vi "AlGaInPAs_v22a.vi"(2 "Debug Mode":bool, 3 "Elapsed Time(s)":dbl, 4 "State":enum16{"Edit", "Start", "Run", "End", "Idle"}(ring), 5 "Argument List In":string[](array[string])) -> (0 "Status Out":string, 1 "Argument List Out":string[](array[string]))   [LabVIEW 2011]
uses:
  high_level_proc/source_dilution.ctl
  high_level_proc/source_noDilution.ctl
panel:
  out "source array":refnum<vi>[](array[refnum])
  in  "Zn bubbler":T1={"Dilution"=FALSE, "Calculated"=0, "MFC1 flow"=0.0, "MFC2 flow"=10.0, "MFC3 flow"=100.0, "Bubbler (main)"={"Flow"=0.0, "Prep"=FALSE, "Run"=FALSE, "Active"=FALSE, "Name"=""}} caption="Al" {"Bubbler (main)"."Flow" format="%.2f"; "MFC1 flow" format="%.4f"; "MFC3 flow" format="%.1f"; "MFC2 flow" format="%.2f"; "Calculated" items=["Flow", "MFC1", "MFC2", "MFC3"]}
  in  "Al bubbler":T2 caption="Al" {"Flow" format="%.2f"}
  in  "Se bubbler":T1={"Dilution"=FALSE, "Calculated"=0, "MFC1 flow"=0.0, "MFC2 flow"=10.0, "MFC3 flow"=100.0, "Bubbler (main)"={"Flow"=0.0, "Prep"=FALSE, "Run"=FALSE, "Active"=FALSE, "Name"="Se"}} caption="Al" {"Bubbler (main)"."Flow" format="%.2f"; "MFC1 flow" format="%.4f"; "MFC3 flow" format="%.1f"; "MFC2 flow" format="%.2f"; "Calculated" items=["Flow", "MFC1", "MFC2", "MFC3"]}
  in  "P bubbler":T2={"Flow"=0.0, "Prep"=FALSE, "Run"=FALSE, "Active"=FALSE, "Name"="P liq"} caption="Al" {"Flow" format="%.2f"}
  in  "As gas":T2={"Flow"=0.0, "Prep"=FALSE, "Run"=FALSE, "Active"=FALSE, "Name"="As gas"} caption="Al" {"Flow" format="%.2f"}
  in  "P gas":T2={"Flow"=0.0, "Prep"=FALSE, "Run"=FALSE, "Active"=FALSE, "Name"="P gas"} caption="Al" {"Flow" format="%.2f"}
  in  "In bubbler":T2 caption="Al" {"Flow" format="%.2f"}
  in  "Ga bubbler":T1={"Dilution"=FALSE, "Calculated"=0, "MFC1 flow"=0.0, "MFC2 flow"=10.0, "MFC3 flow"=100.0, "Bubbler (main)"={"Flow"=0.0, "Prep"=FALSE, "Run"=FALSE, "Active"=FALSE, "Name"=""}} caption="Al" {"Bubbler (main)"."Flow" format="%.2f"; "MFC1 flow" format="%.4f"; "MFC3 flow" format="%.1f"; "MFC2 flow" format="%.2f"; "Calculated" items=["Flow", "MFC1", "MFC2", "MFC3"]}
  out "prep_done":bool
  out "run started":bool
  out "first":bool=TRUE
  out "is OK?":bool
  in  "prep_time":dbl
  in  "Cancel":bool
  in  "OK":bool
  # "s"
  # "Add pre-run time to run time in editor."
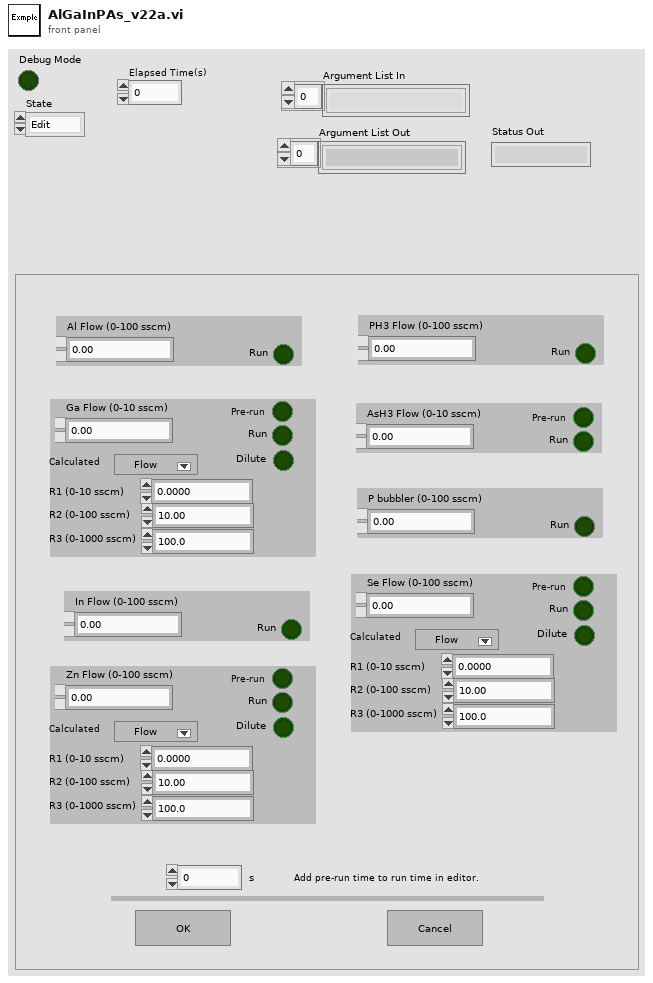
[diagram p1: front panel]
types:
  T1 = typedef "source_dilution.ctl" = cluster{"Dilution":bool, "Calculated":u16, "MFC1 flow":dbl, "MFC2 flow":dbl, "MFC3 flow":dbl, "Bubbler (main)":T2}
  T2 = typedef "source_noDilution.ctl" = cluster{"Flow":dbl, "Prep":bool, "Run":bool, "Active":bool, "Name":string}
  T3 = enum32{"Invalid", "Default", "Floating", "Floating/Auto-Hide", "Modal"}
  T4 = enum16{"Discrete", "Continuous", "Instantaneous", "Finite"}
  T5 = cluster{"Flow":dbl, "Prep":bool, "Run":bool, "Active":bool, "Name":string}
  T6 = cluster{"Dilution":bool, "Calculated":u16, "MFC1 flow":dbl, "MFC2 flow":dbl, "MFC3 flow":dbl, "Bubbler (main)":T2}
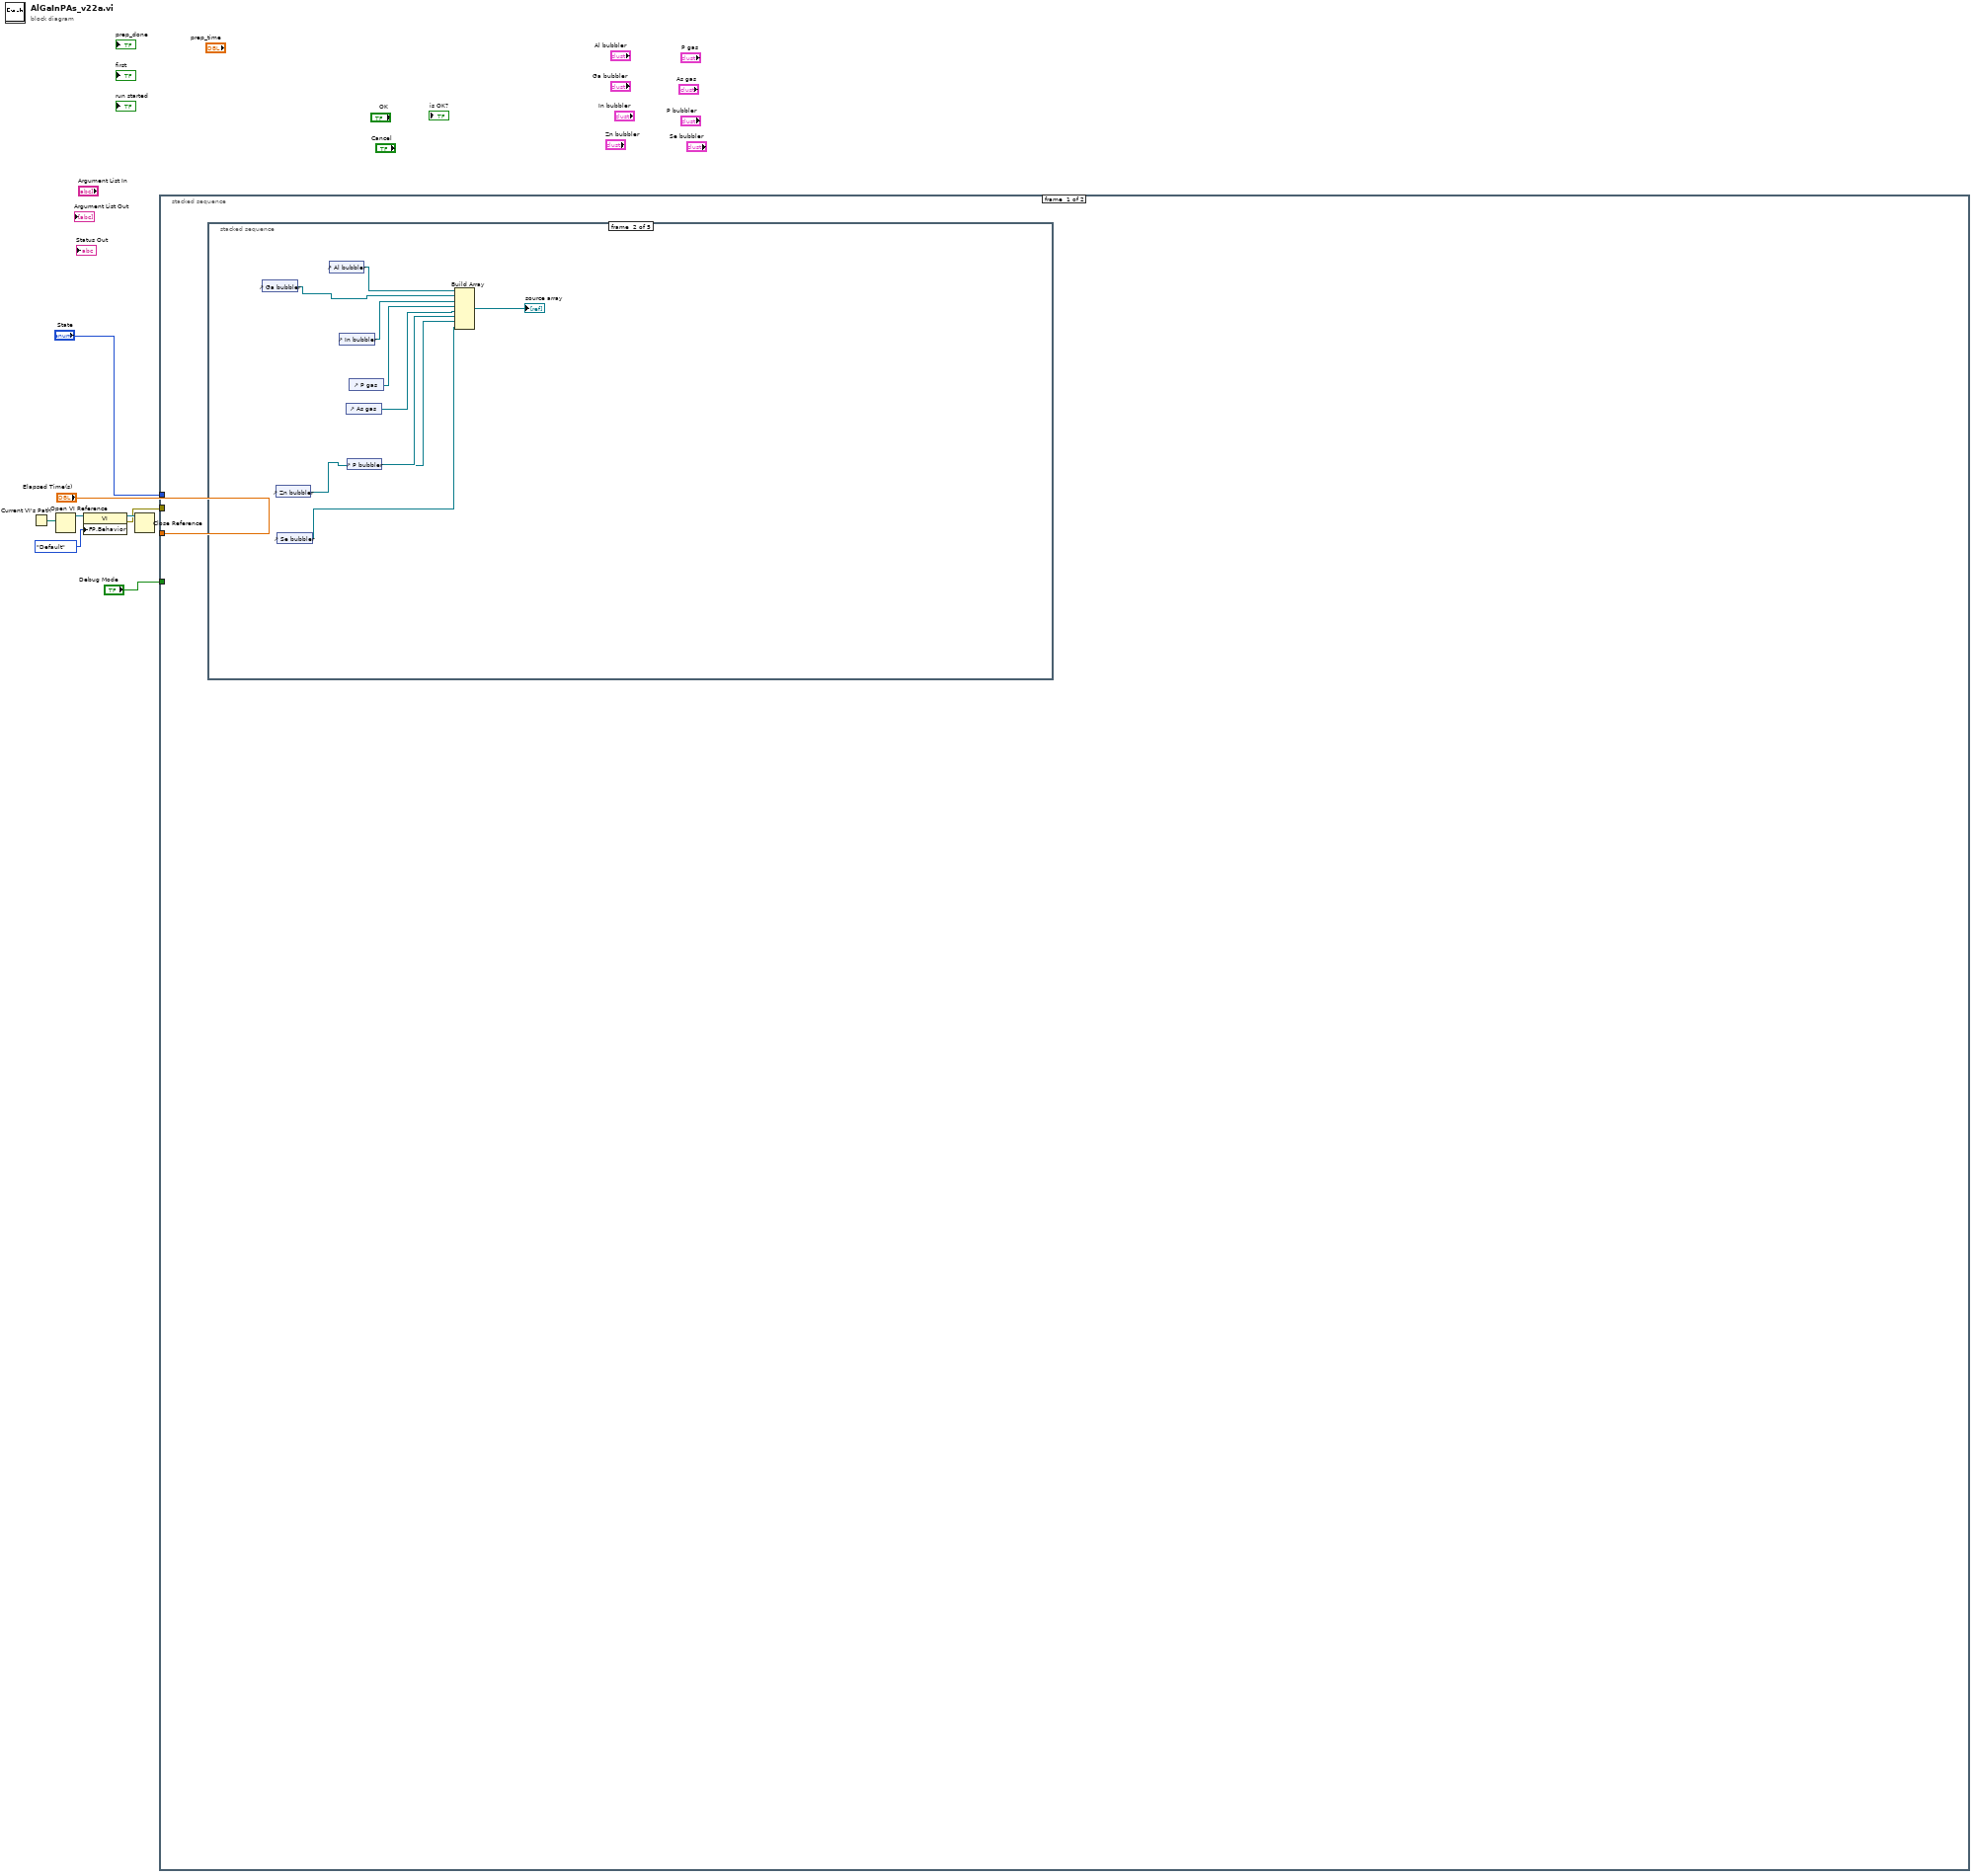
[diagram p0: block diagram]
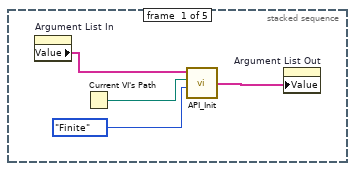
[diagram p2: hidden frame]
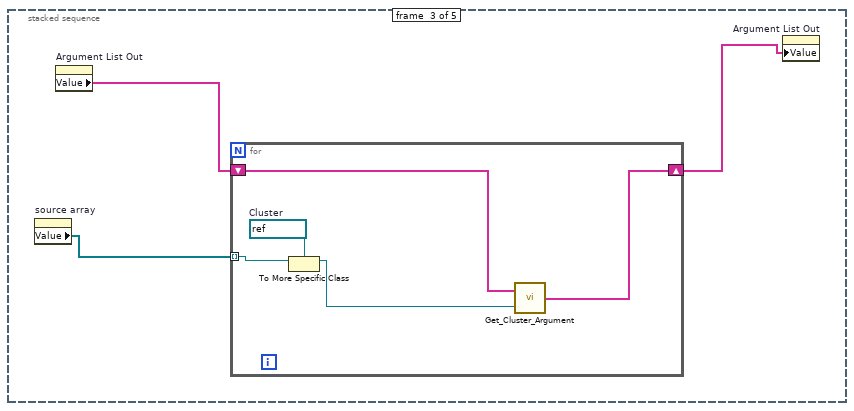
[diagram p3: hidden frame]
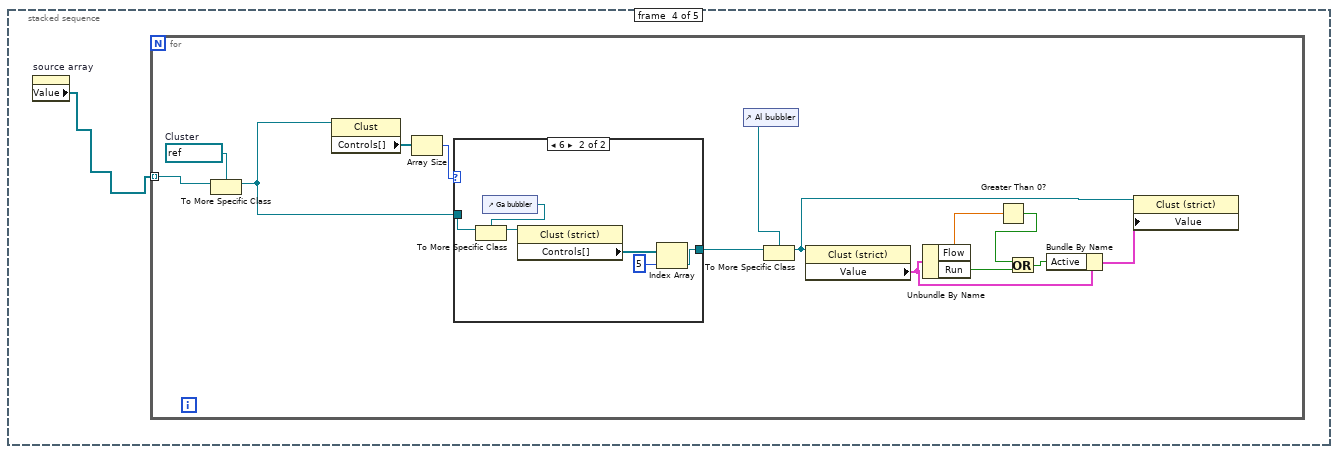
[diagram p4: hidden frame]
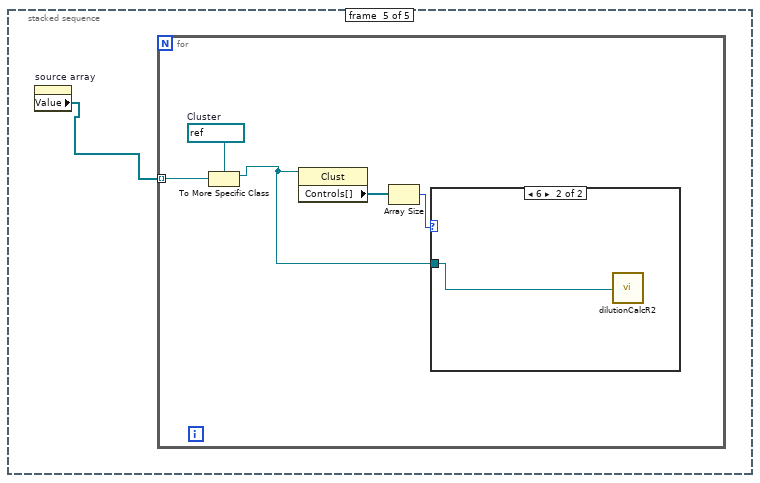
[diagram p6: hidden frame]
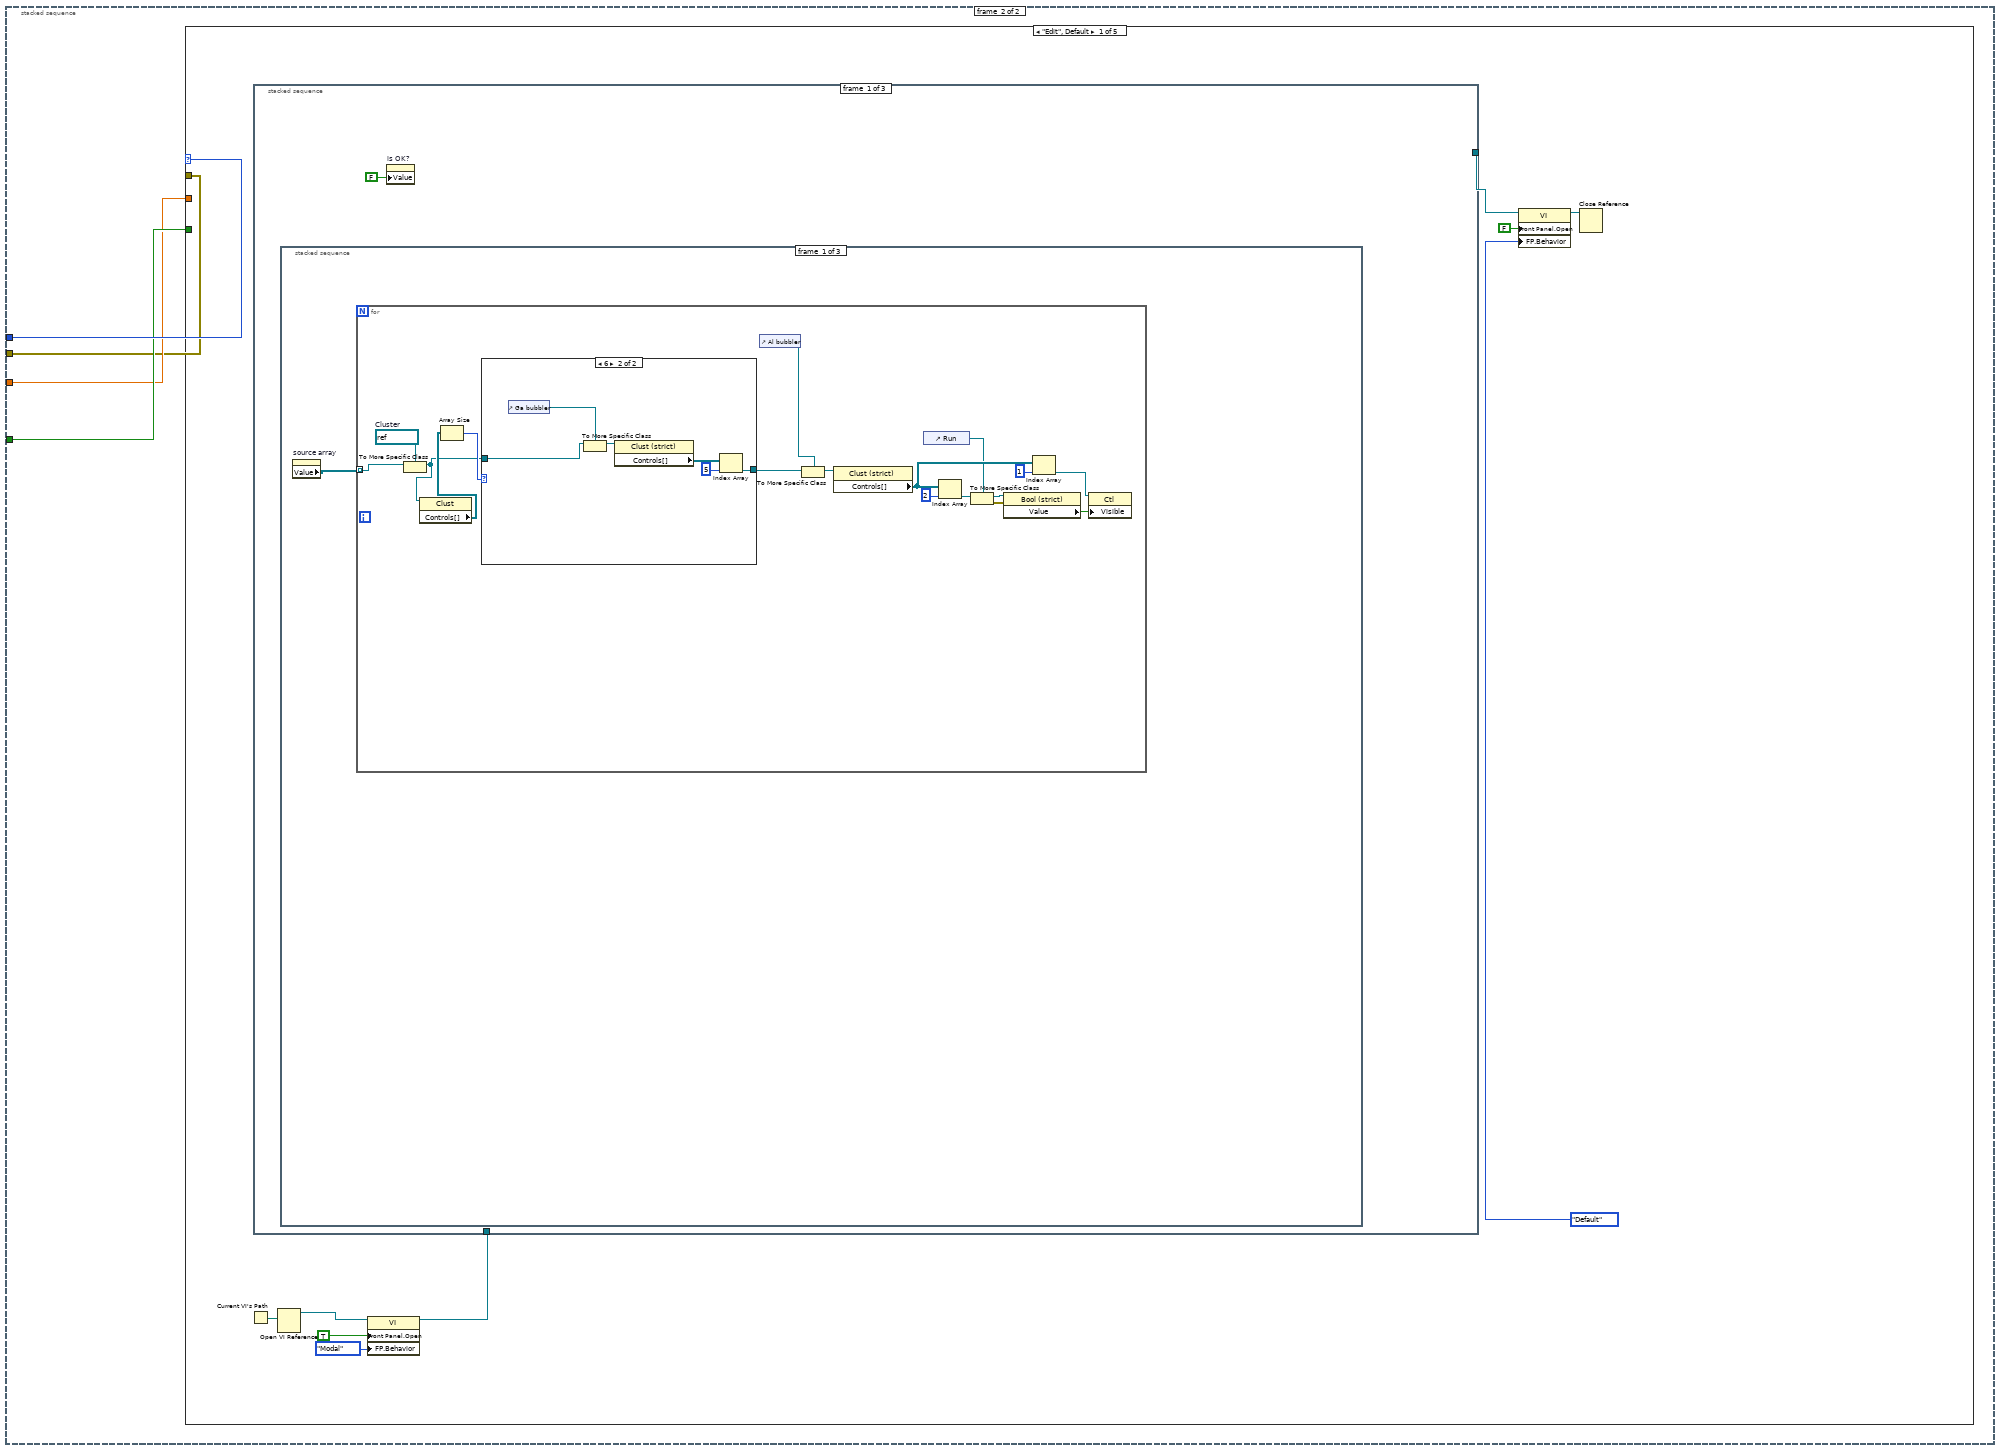
[diagram p8: hidden frame]
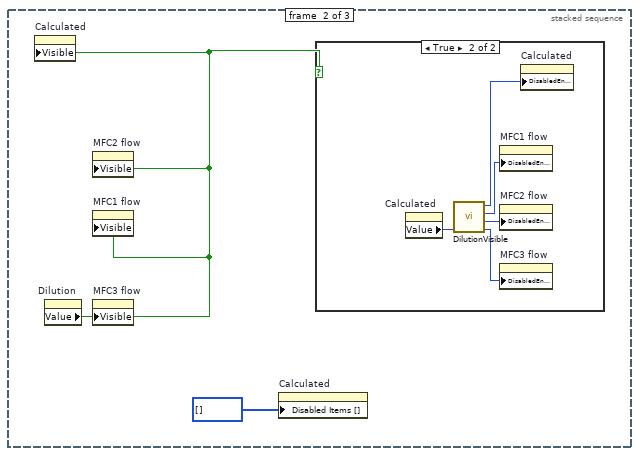
[diagram p10: hidden frame]
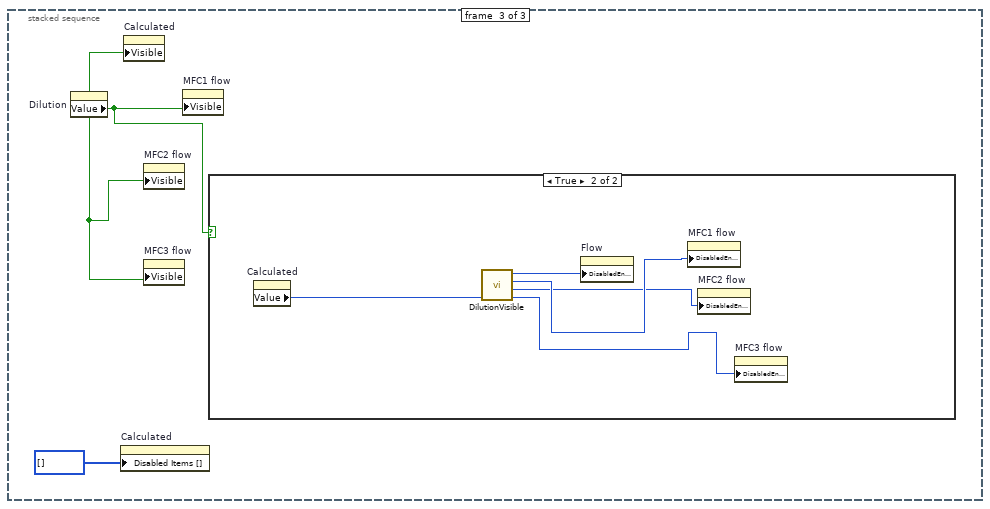
[diagram p12: hidden frame]
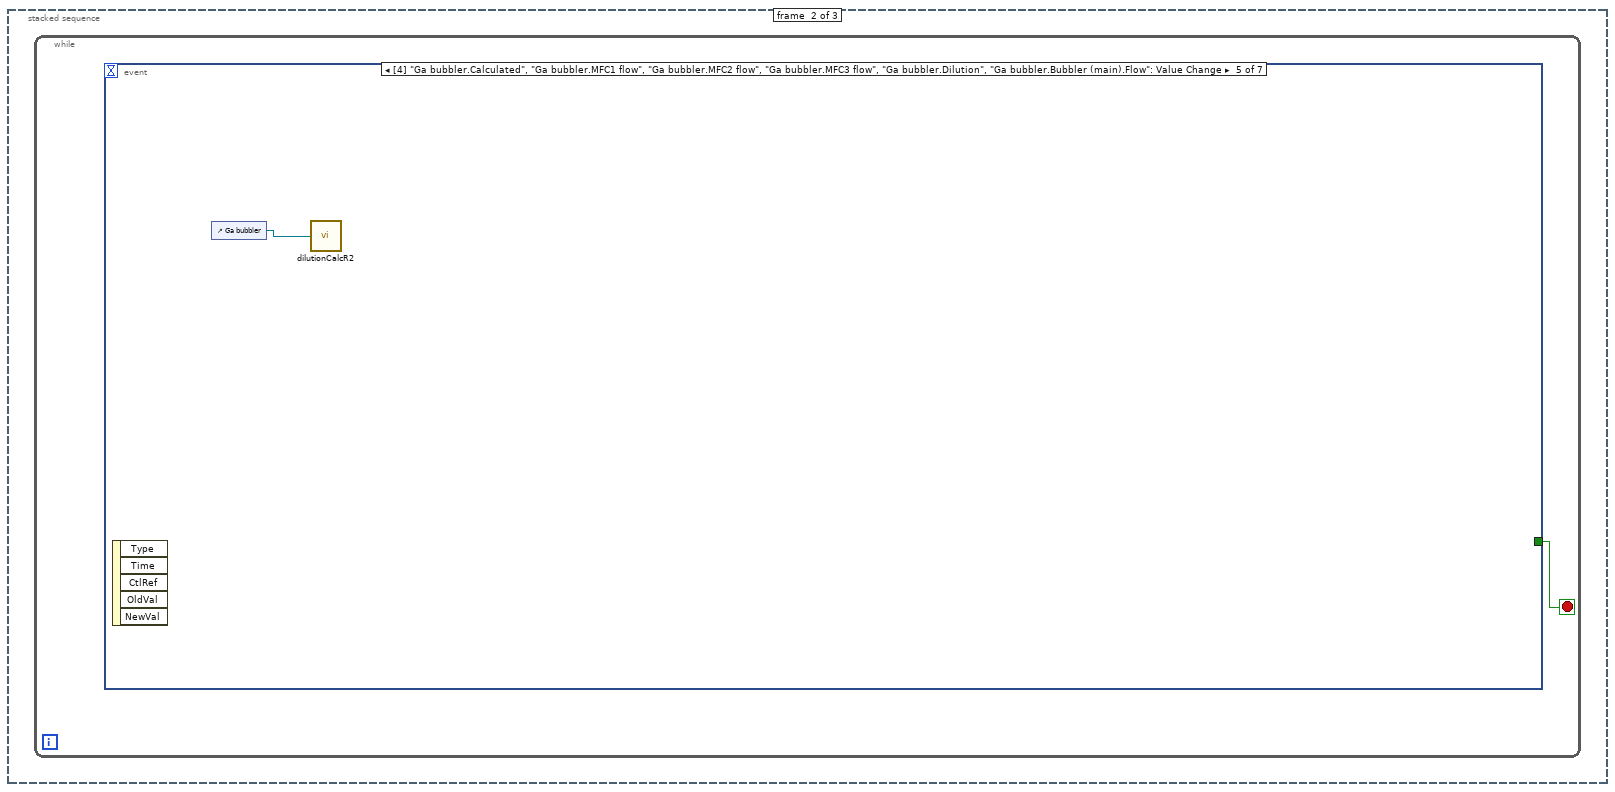
[diagram p14: hidden frame]
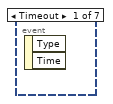
[diagram p15: hidden frame]
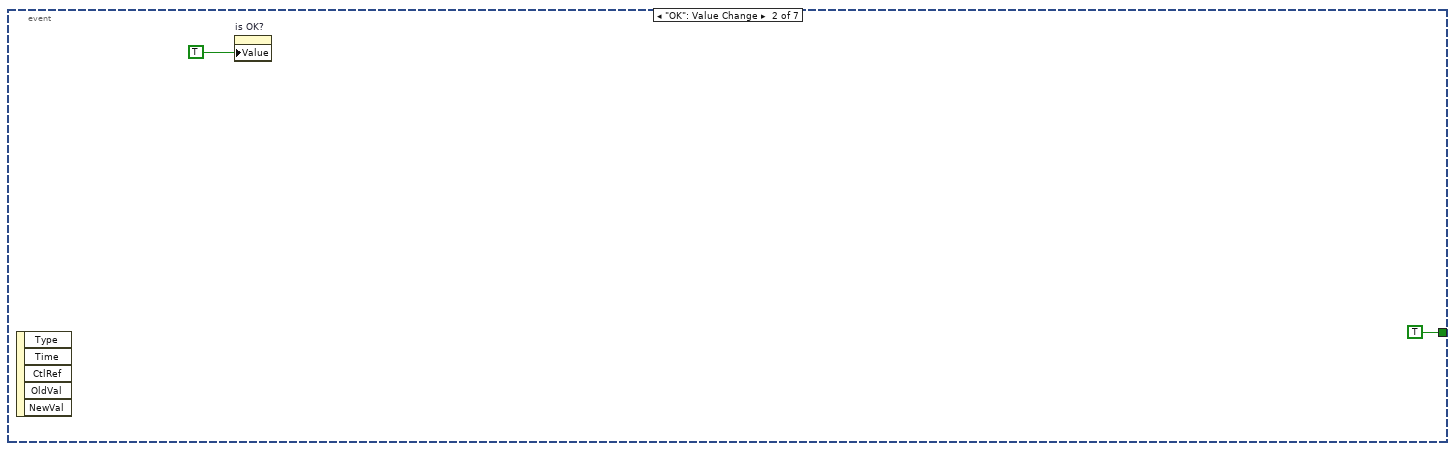
[diagram p16: hidden frame]
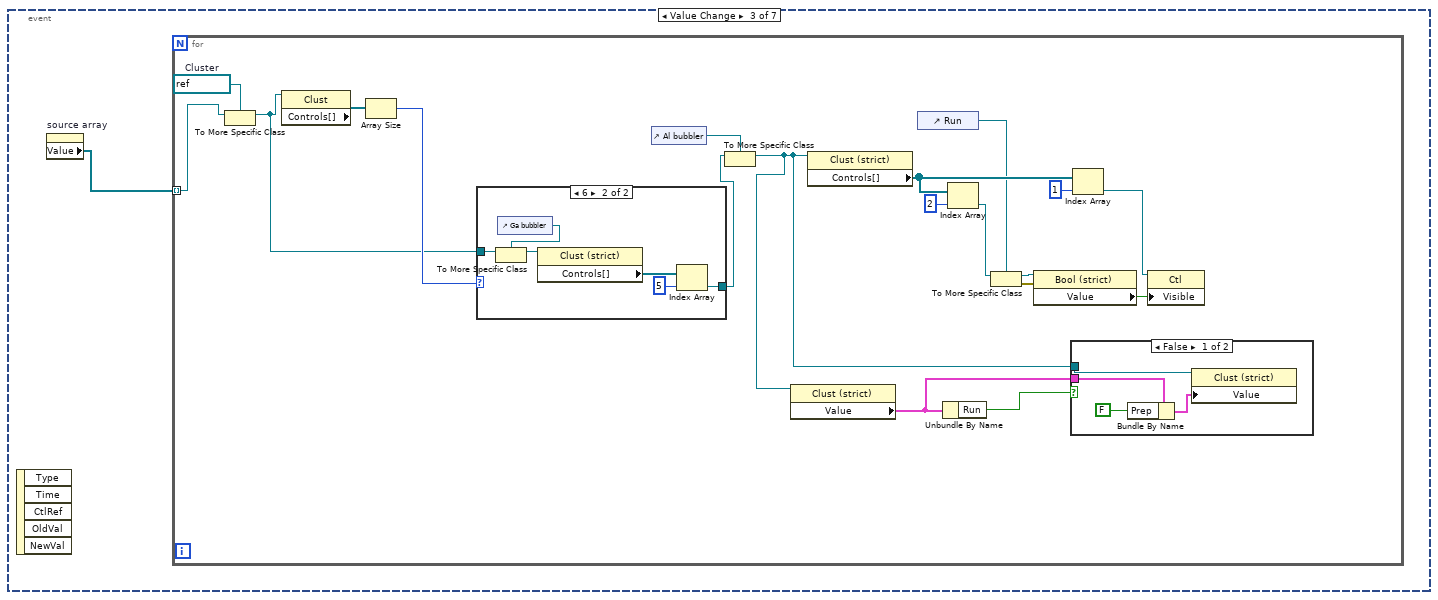
[diagram p17: hidden frame]
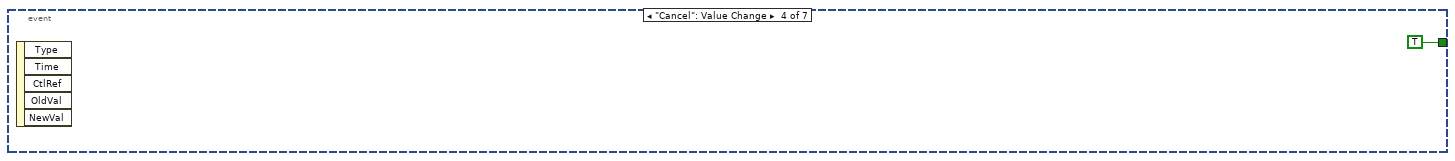
[diagram p20: hidden frame]
diagram:
  n1 = Current VI's Path() -> (path=w5:path)
  n2 = Open VI Reference(vi path=w5) -> (vi reference=w4:refnum<vi>)  [unwired: 1 in, 5 out]
  n3 = property class="VI"(reference=w4, "FP.Behavior"=T3."Default" ("Front Panel Window:Behavior")) -> (reference out=w2:refnum<vi>, error out=w1:errorcluster)  [unwired: 1 in]
  n4 = Close Reference(reference=w2) -> ()  [unwired: 1 in, 1 out]
  n5 = stacked-sequence {
    tunnel: "State" -> [_ w62]
    tunnel: "Debug Mode" -> [_ w61]
    tunnel: "Elapsed Time(s)" -> [_ w60]
    tunnel: w1 -> [_ w59]
    frame #0 {
      n6 = stacked-sequence {
        frame #0 {
          n7 = property on="Argument List In" class="Arr (strict)"() -> ("Value"=w12:string[])  [unwired: 2 in, 2 out]
          n8 = Current VI's Path() -> (path=w9:path)
          n9 = call "API_Init.vi"("API Mode"=T4."Finite", "VI Path"=w9, "Argument List In"=w12) -> ("Argument List Out"=w11:string[])  [unwired: 1 in]
          n10 = property on="Argument List Out" class="Arr (strict)"("Value"=w11) -> ()  [unwired: 2 in, 2 out]
        }
        frame #1 {
          n11 = control-ref of="Ga bubbler"() -> (w16:refnum<vi>)
          n12 = control-ref of="Zn bubbler"() -> (w15:refnum<vi>)
          n13 = control-ref of="Se bubbler"() -> (w14:refnum<vi>)
          n14 = control-ref of="Al bubbler"() -> (w21:refnum<vi>)
          n15 = control-ref of="In bubbler"() -> (w20:refnum<vi>)
          n16 = control-ref of="As gas"() -> (w18:refnum<vi>)
          n17 = control-ref of="P bubbler"() -> (w17:refnum<vi>)
          n18 = control-ref of="P gas"() -> (w19:refnum<vi>)
          n19 = Build Array(w21, w16, w20, w19, w18, w17, w15, w14) -> (→"source array":refnum<vi>[])
        }
        frame #2 {
          n20 = property on="source array" class="Arr (strict)"() -> ("Value"=w22:refnum<vi>[])  [unwired: 2 in, 2 out]
          n21 = property on="Argument List Out" class="Arr (strict)"() -> ("Value"=w24:string[])  [unwired: 2 in, 2 out]
          n22 = for {
            shift-right: [w28] -> w23
            shift-left: w24 -> [w29]
            tunnel: w22 -> [w27] mode=indexing
            w25 = refnum<vi> refnum  # Cluster
            n23 = To More Specific Class(target class=w25, reference=w27) -> (specific class reference=w26:refnum<vi>)  [unwired: 1 in, 1 out]
            n24 = call "Get_Cluster_Argument.vi"("source"=w26, "Argument List In"=w29) -> ("Argument List Out"=w28:string[])
          }
          n25 = property on="Argument List Out" class="Arr (strict)"("Value"=w23) -> ()  [unwired: 2 in, 2 out]
        }
        frame #3 {
          n26 = property on="source array" class="Arr (strict)"() -> ("Value"=w30:refnum<vi>[])  [unwired: 2 in, 2 out]
          n27 = for {
            tunnel: w30 -> [w33] mode=indexing
            w31 = refnum<vi> refnum  # Cluster
            n28 = To More Specific Class(target class=w31, reference=w33) -> (specific class reference=w32:refnum<vi>)  [unwired: 1 in, 1 out]
            n29 = property class="Clust"(reference=w32) -> ("Controls[]"=w35:refnum<vi>[])  [unwired: 1 in, 2 out]
            n30 = Array Size(array=w35) -> (size(s)=w36:i32)
            n31 = case shown="6" w36 {
              tunnel: [w45 w47] -> w34
              tunnel: w32 -> [w45 w50]
              frame Default {
              }
              frame 6 {
                n32 = control-ref of="Ga bubbler"() -> (w46:refnum<vi>)
                n33 = To More Specific Class(target class=w46, reference=w50) -> (specific class reference=w49:refnum<vi>)  [unwired: 1 in, 1 out]
                n34 = property class="Clust (strict)"(reference=w49) -> ("Controls[]"=w48:refnum<vi>[])  [unwired: 1 in, 2 out]
                n35 = Index Array(array=w48, index=5) -> (element=w47:refnum<vi>)
              }
            }
            n36 = control-ref of="Al bubbler"() -> (w38:refnum<vi>)
            n37 = To More Specific Class(target class=w38, reference=w34) -> (specific class reference=w37:refnum<vi>)  [unwired: 1 in, 1 out]
            n38 = property class="Clust (strict)"(reference=w37) -> ("Value"=w41:T5)  [unwired: 1 in, 2 out]
            n39 = Unbundle By Name(w41) -> ("Flow"=w44:dbl, "Run"=w42:bool)
            n40 = Greater Than 0?(x=w44) -> (x > 0?=w43:bool)
            n41 = Or(x=w43, y=w42) -> (x .or. y?=w39:bool)
            n42 = Bundle By Name(cluster=w41, "Active"=w39) -> (w40:T5)
            n43 = property class="Clust (strict)"(reference=w37, "Value"=w40) -> ()  [unwired: 1 in, 2 out]
          }
        }
        frame #4 {
          n44 = property on="source array" class="Arr (strict)"() -> ("Value"=w52:refnum<vi>[])  [unwired: 2 in, 2 out]
          n45 = for {
            tunnel: w52 -> [w56] mode=indexing
            w54 = refnum<vi> refnum  # Cluster
            n46 = To More Specific Class(target class=w54, reference=w56) -> (specific class reference=w55:refnum<vi>)  [unwired: 1 in, 1 out]
            n47 = property class="Clust"(reference=w55) -> ("Controls[]"=w53:refnum<vi>[])  [unwired: 1 in, 2 out]
            n48 = Array Size(array=w53) -> (size(s)=w57:i32)
            n49 = case shown="6" w57 {
              tunnel: w55 -> [_ w58]
              frame Default {
              }
              frame 6 {
                n50 = call "dilutionCalcR2.vi"("Clust Refnum"=w58) -> ()
              }
            }
          }
        }
      }
    }
    frame #1 {
      n51 = case shown="\"Edit\", Default" w62 {
        tunnel: w61 -> [_ w169 w185 _ _]
        tunnel: w60 -> [_ _ w186 _ _]
        tunnel: w59 -> [_ _ _ _ _]
        frame "Edit", Default {
          n52 = Current VI's Path() -> (path=w67:path)
          n53 = Open VI Reference(vi path=w67) -> (vi reference=w66:refnum<vi>)  [unwired: 1 in, 5 out]
          n54 = property class="VI"(reference=w66, "Front Panel.Open"=TRUE ("Front Panel Window:Open"), "FP.Behavior"=T3."Modal" ("Front Panel Window:Behavior")) -> (reference out=w64:refnum<vi>)  [unwired: 1 in, 1 out]
          n55 = stacked-sequence {
            tunnel: [_ _ w152] -> w69
            tunnel: w64 -> [_ _ w152]
            frame #0 {
              n56 = stacked-sequence {
                frame #0 {
                  n57 = property on="source array" class="Arr (strict)"() -> ("Value"=w73:refnum<vi>[])  [unwired: 2 in, 2 out]
                  n58 = for {
                    tunnel: w73 -> [w78] mode=indexing
                    w77 = refnum<vi> refnum  # Cluster
                    n59 = To More Specific Class(target class=w77, reference=w78) -> (specific class reference=w74:refnum<vi>)  [unwired: 1 in, 1 out]
                    n60 = property class="Clust"(reference=w74) -> ("Controls[]"=w76:refnum<vi>[])  [unwired: 1 in, 2 out]
                    n61 = Array Size(array=w76) -> (size(s)=w75:i32)
                    n62 = case shown="6" w75 {
                      tunnel: w74 -> [w91 w94]
                      tunnel: [w91 w95] -> w80
                      frame Default {
                      }
                      frame 6 {
                        n63 = control-ref of="Ga bubbler"() -> (w92:refnum<vi>)
                        n64 = To More Specific Class(target class=w92, reference=w94) -> (specific class reference=w93:refnum<vi>)  [unwired: 1 in, 1 out]
                        n65 = property class="Clust (strict)"(reference=w93) -> ("Controls[]"=w97:refnum<vi>[])  [unwired: 1 in, 2 out]
                        n66 = Index Array(array=w97, index=5) -> (element=w95:refnum<vi>)
                      }
                    }
                    n67 = control-ref of="Al bubbler"() -> (w81:refnum<vi>)
                    n68 = To More Specific Class(target class=w81, reference=w80) -> (specific class reference=w88:refnum<vi>)  [unwired: 1 in, 1 out]
                    n69 = property class="Clust (strict)"(reference=w88) -> ("Controls[]"=w87:refnum<vi>[])  [unwired: 1 in, 2 out]
                    n70 = control-ref of="Run"() -> (w79:refnum<vi>)
                    n71 = Index Array(array=w87, index=2) -> (element=w85:refnum<vi>)
                    n72 = To More Specific Class(target class=w79, reference=w85) -> (specific class reference=w84:refnum<vi>, error out=w83:errorcluster)  [unwired: 1 in]
                    n73 = property class="Bool (strict)"(reference=w84, error in=w83) -> ("Value"=w82:bool)  [unwired: 2 out]
                    n74 = Index Array(array=w87, index=1) -> (element=w89:refnum<vi>)
                    n75 = property class="Ctl"(reference=w89, "Visible"=w82) -> ()  [unwired: 1 in, 2 out]
                  }
                }
                frame #1 {
                  n76 = property on="Dilution" class="Bool (strict)"() -> ("Value"=w99:bool)  [unwired: 2 in, 2 out]
                  n77 = property on="Calculated" class="Ring (strict)"("Visible"=w99) -> ()  [unwired: 2 in, 2 out]
                  n78 = property on="MFC2 flow" class="DigNum (strict)"("Visible"=w99) -> ()  [unwired: 2 in, 2 out]
                  n79 = property on="MFC1 flow" class="DigNum (strict)"("Visible"=w99) -> ()  [unwired: 2 in, 2 out]
                  n80 = property on="MFC3 flow" class="DigNum (strict)"("Visible"=w99) -> ()  [unwired: 2 in, 2 out]
                  n81 = property on="Calculated" class="Ring (strict)"("Disabled Items []"=i32[] []) -> ()  [unwired: 2 in, 2 out]
                  n82 = case shown="True" w99 {
                    frame False {
                    }
                    frame True {
                      n83 = property on="Calculated" class="Ring (strict)"() -> ("Value"=w101:u16)  [unwired: 2 in, 2 out]
                      n84 = call "DilutionVisible.vi"("calculated"=w101) -> ("MFC3"=w104:u16, "MFC2"=w103:u16, "MFC1"=w102:u16, "flow"=w100:u16)  [unwired: 3 in]
                      n85 = property on="MFC1 flow" class="DigNum (strict)"("DisabledEnum"=w102) -> ()  [unwired: 2 in, 2 out]
                      n86 = property on="MFC2 flow" class="DigNum (strict)"("DisabledEnum"=w103) -> ()  [unwired: 2 in, 2 out]
                      n87 = property on="MFC3 flow" class="DigNum (strict)"("DisabledEnum"=w104) -> ()  [unwired: 2 in, 2 out]
                      n88 = property on="Calculated" class="Ring (strict)"("DisabledEnum"=w100) -> ()  [unwired: 2 in, 2 out]
                    }
                  }
                }
                frame #2 {
                  n89 = property on="Dilution" class="Bool (strict)"() -> ("Value"=w105:bool)  [unwired: 2 in, 2 out]
                  n90 = property on="Calculated" class="Ring (strict)"("Disabled Items []"=i32[] []) -> ()  [unwired: 2 in, 2 out]
                  n91 = property on="Calculated" class="Ring (strict)"("Visible"=w105) -> ()  [unwired: 2 in, 2 out]
                  n92 = property on="MFC2 flow" class="DigNum (strict)"("Visible"=w105) -> ()  [unwired: 2 in, 2 out]
                  n93 = property on="MFC3 flow" class="DigNum (strict)"("Visible"=w105) -> ()  [unwired: 2 in, 2 out]
                  n94 = property on="MFC1 flow" class="DigNum (strict)"("Visible"=w105) -> ()  [unwired: 2 in, 2 out]
                  n95 = case shown="True" w105 {
                    frame False {
                    }
                    frame True {
                      n96 = property on="Calculated" class="Ring (strict)"() -> ("Value"=w110:u16)  [unwired: 2 in, 2 out]
                      n97 = call "DilutionVisible.vi"("calculated"=w110) -> ("MFC3"=w108:u16, "MFC2"=w107:u16, "MFC1"=w109:u16, "flow"=w111:u16)  [unwired: 3 in]
                      n98 = property on="Flow" class="DigNum (strict)"("DisabledEnum"=w111) -> ()  [unwired: 2 in, 2 out]
                      n99 = property on="MFC1 flow" class="DigNum (strict)"("DisabledEnum"=w109) -> ()  [unwired: 2 in, 2 out]
                      n100 = property on="MFC2 flow" class="DigNum (strict)"("DisabledEnum"=w107) -> ()  [unwired: 2 in, 2 out]
                      n101 = property on="MFC3 flow" class="DigNum (strict)"("DisabledEnum"=w108) -> ()  [unwired: 2 in, 2 out]
                    }
                  }
                }
              }
              n102 = property on="is OK?" class="Bool (strict)"("Value"=FALSE ("is OK?")) -> ()  [unwired: 2 in, 2 out]
            }
            frame #1 {
              n103 = while {
                stop <- w112 stop-if-true
                n104 = event shown="[4] \"Ga bubbler.Calculated\", \"Ga bubbler.MFC1 flow\", \"Ga bubbler.MFC2 flow\", \"Ga bubbler.MFC3 flow\", \"Ga bubbler.Dilution\", \"Ga bubbler.Bubbler (main).Flow\": Value Change" {
                  selector: _ -> [_ _ _ _ _ _ _]
                  dyn-events: _ -> [_ _ _ _ _ _ _]
                  timeout: _ -> [_ _ _ _ _ _ _]
                  tunnel: [_ TRUE _ TRUE _ _ _] -> w112
                  event Timeout {
                    n105 = event-data() -> ()  [unwired: 1 in, 2 out]
                  }
                  event "OK": Value Change {
                    n106 = event-data() -> ()  [unwired: 1 in, 5 out]
                    n107 = property on="is OK?" class="Bool (strict)"("Value"=TRUE ("is OK?")) -> ()  [unwired: 2 in, 2 out]
                  }
                  event Value Change {
                    n108 = event-data() -> ()  [unwired: 1 in, 5 out]
                    n109 = property on="source array" class="Arr (strict)"() -> ("Value"=w115:refnum<vi>[])  [unwired: 2 in, 2 out]
                    n110 = for {
                      tunnel: w115 -> [w118] mode=indexing
                      w116 = refnum<vi> refnum  # Cluster
                      n111 = To More Specific Class(target class=w116, reference=w118) -> (specific class reference=w117:refnum<vi>)  [unwired: 1 in, 1 out]
                      n112 = property class="Clust"(reference=w117) -> ("Controls[]"=w120:refnum<vi>[])  [unwired: 1 in, 2 out]
                      n113 = Array Size(array=w120) -> (size(s)=w119:i32)
                      n114 = case shown="6" w119 {
                        tunnel: w117 -> [w135 w138]
                        tunnel: [w135 w139] -> w122
                        frame Default {
                        }
                        frame 6 {
                          n115 = control-ref of="Ga bubbler"() -> (w136:refnum<vi>)
                          n116 = To More Specific Class(target class=w136, reference=w138) -> (specific class reference=w137:refnum<vi>)  [unwired: 1 in, 1 out]
                          n117 = property class="Clust (strict)"(reference=w137) -> ("Controls[]"=w141:refnum<vi>[])  [unwired: 1 in, 2 out]
                          n118 = Index Array(array=w141, index=5) -> (element=w139:refnum<vi>)
                        }
                      }
                      n119 = control-ref of="Al bubbler"() -> (w126:refnum<vi>)
                      n120 = To More Specific Class(target class=w126, reference=w122) -> (specific class reference=w123:refnum<vi>)  [unwired: 1 in, 1 out]
                      n121 = property class="Clust (strict)"(reference=w123) -> ("Value"=w125:T5)  [unwired: 1 in, 2 out]
                      n122 = property class="Clust (strict)"(reference=w123) -> ("Controls[]"=w132:refnum<vi>[])  [unwired: 1 in, 2 out]
                      n123 = control-ref of="Run"() -> (w121:refnum<vi>)
                      n124 = Unbundle By Name(w125) -> ("Run"=w124:bool)
                      n125 = Index Array(array=w132, index=2) -> (element=w130:refnum<vi>)
                      n126 = To More Specific Class(target class=w121, reference=w130) -> (specific class reference=w129:refnum<vi>, error out=w128:errorcluster)  [unwired: 1 in]
                      n127 = property class="Bool (strict)"(reference=w129, error in=w128) -> ("Value"=w127:bool)  [unwired: 2 out]
                      n128 = case shown="False" w124 {
                        tunnel: w125 -> [w145 _]
                        tunnel: w123 -> [w142 _]
                        frame False {
                          n129 = Bundle By Name(cluster=w145, "Prep"=FALSE) -> (w143:T5)
                          n130 = property class="Clust (strict)"(reference=w142, "Value"=w143) -> ()  [unwired: 1 in, 2 out]
                        }
                        frame True {
                        }
                      }
                      n131 = Index Array(array=w132, index=1) -> (element=w133:refnum<vi>)
                      n132 = property class="Ctl"(reference=w133, "Visible"=w127) -> ()  [unwired: 1 in, 2 out]
                    }
                  }
                  event "Cancel": Value Change {
                    n133 = event-data() -> ()  [unwired: 1 in, 5 out]
                  }
                  event Value Change {
                    n134 = event-data() -> ()  [unwired: 1 in, 5 out]
                    n135 = control-ref of="Ga bubbler"() -> (w147:refnum<vi>)
                    n136 = call "dilutionCalcR2.vi"("Clust Refnum"=w147) -> ()
                  }
                  event Value Change {
                    n137 = event-data() -> ()  [unwired: 1 in, 5 out]
                    n138 = control-ref of="Se bubbler"() -> (w148:refnum<vi>)
                    n139 = call "dilutionCalcR2.vi"("Clust Refnum"=w148) -> ()
                  }
                  event Value Change {
                    n140 = event-data() -> ()  [unwired: 1 in, 5 out]
                    n141 = control-ref of="Zn bubbler"() -> (w149:refnum<vi>)
                    n142 = call "dilutionCalcR2.vi"("Clust Refnum"=w149) -> ()
                  }
                }
              }
            }
            frame #2 {
              n143 = property on="Argument List Out" class="Arr (strict)"() -> ("Value"=w151:string[])  [unwired: 2 in, 2 out]
              n144 = property on="is OK?" class="Bool (strict)"() -> ("Value"=w153:bool)  [unwired: 2 in, 2 out]
              n145 = case shown="True" w153 {
                tunnel: w151 -> [w157 w160]
                tunnel: [w157 w159] -> w154
                frame False {
                }
                frame True {
                  n146 = property on="source array" class="Arr (strict)"() -> ("Value"=w158:refnum<vi>[])  [unwired: 2 in, 2 out]
                  n147 = for {
                    shift-right: [w164] -> w159
                    shift-left: w160 -> [w165]
                    tunnel: w158 -> [w163] mode=indexing
                    w162 = refnum<vi> refnum  # Cluster
                    n148 = To More Specific Class(target class=w162, reference=w163) -> (specific class reference=w161:refnum<vi>)  [unwired: 1 in, 1 out]
                    n149 = call "Set_Cluster_Argument.vi"("Clust Refnum"=w161, "Argument List In"=w165) -> ("Argument List Out"=w164:string[])
                  }
                }
              }
              n150 = Current VI's Path() -> (path=w155:path)
              n151 = Not(x=w153) -> (.not. x?=w156:bool)
              n152 = call "API_Edit.vi"("Cancel"=w156, "OK"=w153, "VI Path"=w155, "Argument List In"=w154) -> ("Argument List Out"=w150:string[])
              n153 = property on="Argument List Out" class="Arr (strict)"("Value"=w150) -> ()  [unwired: 2 in, 2 out]
            }
          }
          n154 = property class="VI"(reference=w69, "Front Panel.Open"=FALSE ("Front Panel Window:Open"), "FP.Behavior"=T3."Default" ("Front Panel Window:Behavior")) -> (reference out=w70:refnum<vi>)  [unwired: 1 in, 1 out]
          n155 = Close Reference(reference=w70) -> ()  [unwired: 1 in, 1 out]
        }
        frame "Start" {
          n156 = property on="prep_time" class="DigNum (strict)"() -> ("Value"=w172:dbl)  [unwired: 2 in, 2 out]
          n157 = Greater Than 0?(x=w172) -> (x > 0?=w171:bool)
          n158 = Not(x=w169) -> (.not. x?=w168:bool)
          n159 = property on="Argument List Out" class="Arr (strict)"() -> ("Value"=w167:string[])  [unwired: 2 in, 2 out]
          n160 = And(x=w168, y=w171) -> (x .and. y?=w170:bool)
          n161 = call "Set_Argument.vi"("Enable"=FALSE, "Argument"="run_started", "Argument List In"=w167) -> ("Argument List Out"=w166:string[])
          n162 = case shown="True" w170 {
            frame False {
            }
            frame True {
              n163 = property on="Ga bubbler" class="Clust (strict)"() -> ("Value"=w181:T6)  [unwired: 2 in, 2 out]
              n164 = property on="Zn bubbler" class="Clust (strict)"() -> ("Value"=w175:T6)  [unwired: 2 in, 2 out]
              n165 = property on="Al bubbler" class="Clust (strict)"() -> ("Value"=w182:T5)  [unwired: 2 in, 2 out]
              n166 = property on="In bubbler" class="Clust (strict)"() -> ("Value"=w180:T5)  [unwired: 2 in, 2 out]
              n167 = property on="P gas" class="Clust (strict)"() -> ("Value"=w179:T5)  [unwired: 2 in, 2 out]
              n168 = property on="Se bubbler" class="Clust (strict)"() -> ("Value"=w176:T6)  [unwired: 2 in, 2 out]
              n169 = property on="As gas" class="Clust (strict)"() -> ("Value"=w178:T5)  [unwired: 2 in, 2 out]
              n170 = property on="P bubbler" class="Clust (strict)"() -> ("Value"=w177:T5)  [unwired: 2 in, 2 out]
              n171 = call "Set_V_III.vi"("Se bubbler"=w176, "P bubbler"=w177, "As gas"=w178, "P gas"=w179, "Run Started"=FALSE, "Zn bubbler"=w175, "In bubbler"=w180, "Ga bubbler"=w181, "Al bubbler"=w182) -> ()  [unwired: 3 in]
            }
          }
          n172 = property on="Argument List Out" class="Arr (strict)"("Value"=w166) -> ()  [unwired: 2 in, 2 out]
        }
        frame "Run" {
          n173 = property on="source array" class="Arr (strict)"() -> ("Value"=w184:refnum<vi>[])  [unwired: 2 in, 2 out]
          n174 = stacked-sequence {
            tunnel: w186 -> [_ w191 _ _]
            tunnel: w185 -> [_ _ _ w223]
            tunnel: w184 -> [_ _ w193 _]
            frame #0 {
              n175 = property on="Argument List Out" class="Arr (strict)"() -> ("Value"=w188:string[])  [unwired: 2 in, 2 out]
              n176 = call "Get_Argument.vi"("Argument"="run_started", "Argument List"=w188) -> ("Enabled"=w187:bool)
              n177 = property on="run started" class="Bool (strict)"("Value"=w187) -> ()  [unwired: 2 in, 2 out]
            }
            frame #1 {
              n178 = property on="prep_time" class="DigNum (strict)"() -> ("Value"=w192:dbl)  [unwired: 2 in, 2 out]
              n179 = Greater Or Equal?(x=w191, y=w192) -> (x >= y?=w190:bool)
              n180 = property on="prep_done" class="Bool (strict)"("Value"=w190) -> ()  [unwired: 2 in, 2 out]
            }
            frame #2 {
              n181 = property on="run started" class="Bool (strict)"() -> ("Value"=w194:bool)  [unwired: 2 in, 2 out]
              n182 = Not(x=w194) -> (.not. x?=w196:bool)
              n183 = for {
                shift-right: [w208] -> _
                shift-left: TRUE ("first") -> [w205]
                tunnel: w196 -> [w206]
                tunnel: w193 -> [w199] mode=indexing
                w198 = refnum<vi> refnum  # Cluster
                n184 = To More Specific Class(target class=w198, reference=w199) -> (specific class reference=w197:refnum<vi>)  [unwired: 1 in, 1 out]
                n185 = property class="Clust"(reference=w197) -> ("Controls[]"=w201:refnum<vi>[])  [unwired: 1 in, 2 out]
                n186 = Array Size(array=w201) -> (size(s)=w200:i32)
                n187 = case shown="6" w200 {
                  tunnel: [w215 w218] -> w203
                  tunnel: w197 -> [w215 w216]
                  frame Default {
                  }
                  frame 6 {
                    n188 = control-ref of="Ga bubbler"() -> (w217:refnum<vi>)
                    n189 = To More Specific Class(target class=w217, reference=w216) -> (specific class reference=w221:refnum<vi>)  [unwired: 1 in, 1 out]
                    n190 = property class="Clust (strict)"(reference=w221) -> ("Controls[]"=w220:refnum<vi>[])  [unwired: 1 in, 2 out]
                    n191 = Index Array(array=w220, index=5) -> (element=w218:refnum<vi>)
                  }
                }
                n192 = control-ref of="Al bubbler"() -> (w204:refnum<vi>)
                n193 = To More Specific Class(target class=w204, reference=w203) -> (specific class reference=w202:refnum<vi>)  [unwired: 1 in, 1 out]
                n194 = property class="Clust (strict)"(reference=w202) -> ("Value"=w214:T5)  [unwired: 1 in, 2 out]
                n195 = Unbundle By Name(w214) -> ("Prep"=w213:bool, "Run"=w212:bool, "Active"=w211:bool, "Name"=w207:string)
                n196 = property on="Status Out" class="Str"() -> ("Value"=w210:string)  [unwired: 2 in, 2 out]
                n197 = call "flow_strings.vi"("string in"=w210, "is first in?"=w205, "use source?"=w211, "name"=w207, "run source?"=w212, "prep source?"=w213, "is prep?"=w206) -> ("string out"=w209:string, "is first out?"=w208:bool)
                n198 = property on="Status Out" class="Str"("Value"=w209) -> ()  [unwired: 2 in, 2 out]
              }
            }
            frame #3 {
              n199 = property on="run started" class="Bool (strict)"() -> ("Value"=w225:bool)  [unwired: 2 in, 2 out]
              n200 = Not(x=w225) -> (.not. x?=w224:bool)
              n201 = property on="prep_done" class="Bool (strict)"() -> ("Value"=w226:bool)  [unwired: 2 in, 2 out]
              n202 = And(x=w226, y=w224) -> (x .and. y?=w222:bool)
              n203 = case shown="True" w222 {
                selector: w222 -> [_ w227]
                tunnel: w223 -> [_ w228]
                frame False {
                }
                frame True {
                  n204 = stacked-sequence {
                    tunnel: w228 -> [w230 _]
                    tunnel: w227 -> [w229 _]
                    frame #0 {
                      n205 = case shown="False" w230 {
                        tunnel: w229 -> [w239 _]
                        frame False {
                          n206 = property on="Ga bubbler" class="Clust (strict)"() -> ("Value"=w237:T6)  [unwired: 2 in, 2 out]
                          n207 = property on="In bubbler" class="Clust (strict)"() -> ("Value"=w236:T5)  [unwired: 2 in, 2 out]
                          n208 = property on="P gas" class="Clust (strict)"() -> ("Value"=w235:T5)  [unwired: 2 in, 2 out]
                          n209 = property on="Al bubbler" class="Clust (strict)"() -> ("Value"=w238:T5)  [unwired: 2 in, 2 out]
                          n210 = property on="Zn bubbler" class="Clust (strict)"() -> ("Value"=w231:T6)  [unwired: 2 in, 2 out]
                          n211 = property on="Se bubbler" class="Clust (strict)"() -> ("Value"=w232:T6)  [unwired: 2 in, 2 out]
                          n212 = property on="As gas" class="Clust (strict)"() -> ("Value"=w234:T5)  [unwired: 2 in, 2 out]
                          n213 = property on="P bubbler" class="Clust (strict)"() -> ("Value"=w233:T5)  [unwired: 2 in, 2 out]
                          n214 = call "Set_V_III.vi"("Se bubbler"=w232, "P bubbler"=w233, "As gas"=w234, "P gas"=w235, "Run Started"=w239, "Zn bubbler"=w231, "In bubbler"=w236, "Ga bubbler"=w237, "Al bubbler"=w238) -> ()  [unwired: 3 in]
                        }
                        frame True {
                        }
                      }
                    }
                    frame #1 {
                      n215 = property on="Argument List Out" class="Arr (strict)"() -> ("Value"=w240:string[])  [unwired: 2 in, 2 out]
                      n216 = call "Set_Argument.vi"("Enable"=TRUE, "Argument"="run_started", "Argument List In"=w240) -> ("Argument List Out"=w241:string[])
                      n217 = property on="Argument List Out" class="Arr (strict)"("Value"=w241) -> ()  [unwired: 2 in, 2 out]
                    }
                  }
                }
              }
            }
          }
        }
        frame "End" {
        }
        frame "Idle" {
        }
      }
    }
  }
